vi "getValuesDbl.vi"(8 "error in":errorcluster, 9 "timeout in ms (-1)":i32=100, 11 "notifiers in":refnum<notifier>[](array[refnum])) -> (0 "error out":errorcluster, 2 "notifier values":string[](array[string]), 3 "notifier names":string[](array[string]))   [LabVIEW 2013]
doc: "Takes an array of notifiers and returns two arrays containing the name and value of each notifier. All values have been flattened to strings.\nNotifier value must be a double.\n\nKaitlin Gallagher\n3/4/14"
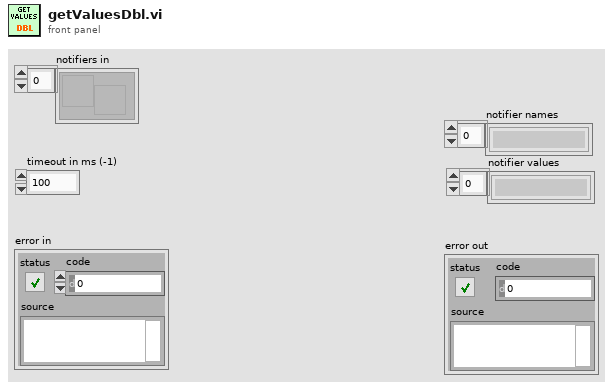
[diagram p1: front panel]
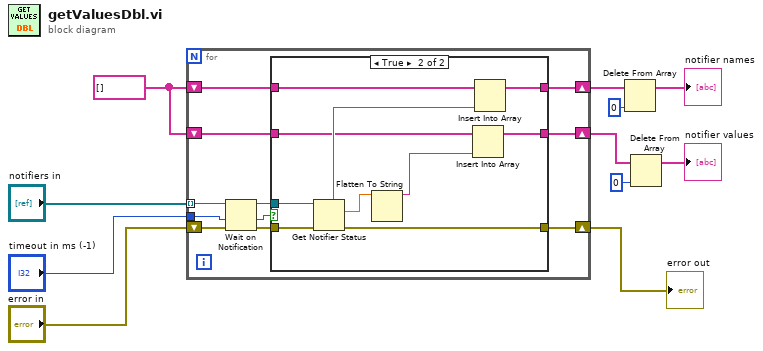
[diagram p0: block diagram]
diagram:
  w1 = string[] [] ("notifier names 2")
  n1 = for {
    tunnel: "notifiers in" -> [w21] mode=indexing
    shift-right: [w22] -> w9
    shift-left: "error in" -> [w19]
    tunnel: "timeout in ms (-1)" -> [w17]
    shift-right: [w14] -> w7
    shift-left: w1 -> [w15]
    shift-right: [w12] -> w4
    shift-left: w1 -> [w13]
    n2 = Wait on Notification(notifier=w21, timeout in ms (-1)=w17, error in (no error)=w19) -> (notifier out=w20:refnum<notifier>, timed out?=w16:bool, error out=w18:errorcluster)  [unwired: 1 in, 1 out]
    n3 = case shown="True" w16 {
      tunnel: [w25 w35] -> w22
      tunnel: w20 -> [_ w33]
      tunnel: w18 -> [w25 w32]
      tunnel: w15 -> [w24 w31]
      tunnel: [w24 w30] -> w14
      tunnel: w13 -> [w23 w27]
      tunnel: [w23 w26] -> w12
      frame False {
      }
      frame True {
        n4 = Get Notifier Status(notifier=w33, error in (no error)=w32) -> (notifier name=w29:string, current notification=w34:dbl, error out=w35:errorcluster)  [unwired: 2 out]
        n5 = Flatten To String(anything=w34) -> (data string=w28:string)  [unwired: 3 in, 2 out]
        n6 = Insert Into Array(array=w27, new element=w28) -> (w26:string[])  [unwired: 1 in]
        n7 = Insert Into Array(array=w31, new element=w29) -> (w30:string[])  [unwired: 1 in]
      }
    }
  }
  "error out" <- w9
  n8 = Delete From Array(array=w7, index=0) -> (array with subset deleted=→"notifier names":string[])  [unwired: 1 in, 1 out]
  n9 = Delete From Array(array=w4, index=0) -> (array with subset deleted=→"notifier values":string[])  [unwired: 1 in, 1 out]
